vi "Place Fruit.vi"(8 "error in (no error)":errorcluster, 11 "Game Board in":refnum<class "Game Board.lvclass">) -> (0 "error out":errorcluster, 3 "Game Board out":refnum<class "Game Board.lvclass">)   [LabVIEW 2020, in "Game Board.lvclass"]
uses:
  Game Board.lvclass
  Game Board.lvclass/Game Board.ctl
  Snake/Type Defs/Coordinates.ctl
  Fruit/Fruit.lvclass
  Snake/Snake.lvclass
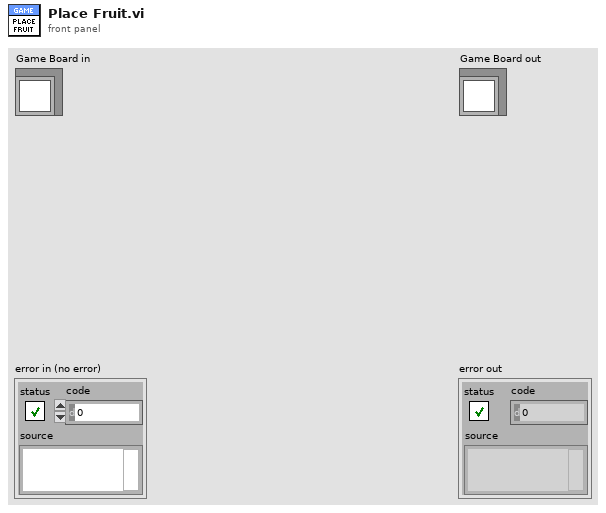
[diagram p1: front panel]
types:
  T1 = typedef "Coordinates.ctl" = cluster{"X":i32, "Y":i32}
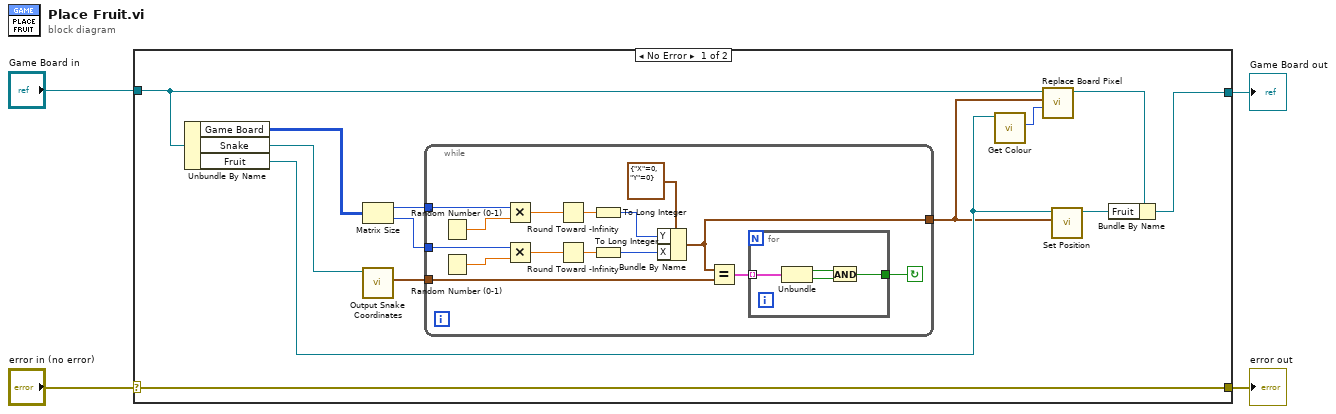
[diagram p0: block diagram]
diagram:
  n1 = case shown="No Error" "error in (no error)" {
    selector: "error in (no error)" -> [w17 w38]
    tunnel: [w17 w38] -> w3
    tunnel: [w15 w37] -> w1
    tunnel: "Game Board in" -> [w8 w37]
    frame No Error {
      n2 = Unbundle By Name(w8) -> ("Game Board"=w16:u32[][], "Snake"=w14:refnum<class "Snake.lvclass">, "Fruit"=w10:refnum<class "Fruit.lvclass">)
      n3 = Matrix Size(0:w16) -> (1:w12:i32, 2:w11:i32)
      n4 = call "Output Snake Coordinates.vi"("Snake in"=w14) -> ("Tail"=w13:T1[])  [unwired: 10 in]
      n5 = while {
        tunnel: w11 -> [w25]
        tunnel: w12 -> [w24]
        tunnel: [w18] -> w6
        tunnel: w13 -> [w22]
        stop <- w23 continue-if-true
        n6 = Random Number (0-1)() -> (number: 0 to 1=w32:dbl)
        n7 = Random Number (0-1)() -> (number: 0 to 1=w31:dbl)
        n8 = Multiply(x=w24, y=w32) -> (x*y=w30:dbl)
        n9 = Multiply(x=w25, y=w31) -> (x*y=w29:dbl)
        n10 = Round Toward -Infinity(1:w30) -> (0:w27:dbl)
        n11 = Round Toward -Infinity(1:w29) -> (0:w28:dbl)
        n12 = To Long Integer(number=w27) -> (32bit integer=w20:i32)
        n13 = To Long Integer(number=w28) -> (32bit integer=w19:i32)
        n14 = Bundle By Name(cluster=T1 {"X"=0, "Y"=0} ("Coordinates"), "Y"=w20, "X"=w19) -> (w18:T1)
        n15 = Equal?(x=w18, y=w22) -> (x = y?=w26:cluster{"X":bool, "Y":bool}[])
        n16 = for {
          tunnel: w26 -> [w36] mode=indexing
          tunnel: [w33] -> w23
          n17 = Unbundle(w36) -> ("X"=w35:bool, "Y"=w34:bool)
          n18 = And(x=w35, y=w34) -> (x .and. y?=w33:bool)
        }
      }
      n19 = call-dynamic "Get Colour.vi"("Game Componants in"=w10) -> ("Componant Colour"=w5:u32)  [unwired: 10 in]
      n20 = call "Replace Board Pixel.vi"("Colour"=w5, "Coordinates"=w6, "Game Board in"=w8) -> ("Game Board out"=w7:refnum<class "Game Board.lvclass">)  [unwired: 7 in, 1 out]
      n21 = call-dynamic "Set Position.vi"("Coordinates"=w6, "Fruit in"=w10) -> ("Fruit out"=w9:refnum<class "Fruit.lvclass">)  [unwired: 9 in]
      n22 = Bundle By Name(cluster=w7, "Fruit"=w9) -> (w15:refnum<class "Game Board.lvclass">)
    }
    frame Error {
    }
  }
  "error out" <- w3
  "Game Board out" <- w1
